vi "Update Schedule.vi"(8 "error in (no error)":errorcluster, 10 "New Schedule":string[](array[string]), 11 "Major Frame in":refnum<class "Major Frame.lvclass">) -> (0 "error out":errorcluster, 2 "Previous Schedule":string[](array[string]), 3 "Major Frame out":refnum<class "Major Frame.lvclass">)   [LabVIEW 2020, in "BCI-1553 API.lvlib" / "Major Frame.lvclass"]
doc: "A method for modifying the schedule contained in a Major Frame. The Schedule is a an array of strings that is already filled with the exact execution order of Minor Frame IDs and Message IDs. This method will return the previous schedule that was in use."
uses:
  Major Frame.lvclass
  Major Frame.lvclass/Major Frame.ctl
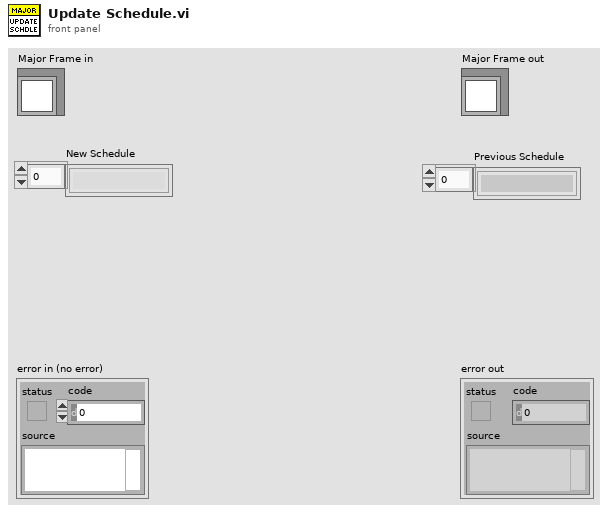
[diagram p1: front panel]
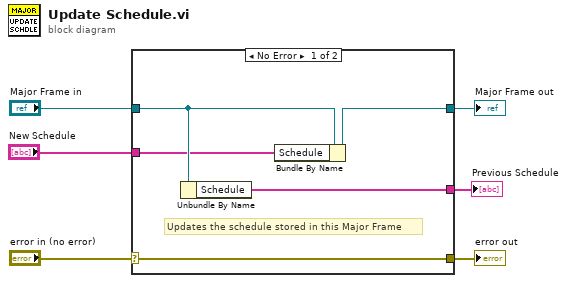
[diagram p0: block diagram]
diagram:
  n1 = case shown="No Error" "error in (no error)" {
    selector: "error in (no error)" -> [w11 w13]
    tunnel: [w11 w13] -> w5
    tunnel: [w9 w12] -> w3
    tunnel: "Major Frame in" -> [w10 w12]
    tunnel: [w8 _] -> w1
    tunnel: "New Schedule" -> [w7 _]
    frame No Error {
      # "Updates the schedule stored in this Major Frame"
      n2 = Unbundle By Name(w10) -> ("Schedule"=w8:string[])
      n3 = Bundle By Name(cluster=w10, "Schedule"=w7) -> (w9:refnum<class "Major Frame.lvclass">)
    }
    frame Error {
    }
  }
  "error out" <- w5
  "Major Frame out" <- w3
  "Previous Schedule" <- w1
